vi "Van Der Pauw Test.vi"(8 "error in (no error)":errorcluster) -> (0 "error out":errorcluster)   [LabVIEW 2016, in "Hall Effect Library.lvlib"]
doc: "This VI executes the Van Der Pauw Resisitivty Test and returns the voltage measurements V1-V8 taken during the test."
uses:
  Hall Effect Library.lvlib
  Controls/Measurement.ctl
  Public/Controls/Data Items.ctl
  Public/Controls/Tests.ctl
  Global Variables/Test Settings.vi
  Global Variables/Instrument Locations.vi
  Global Variables/Hall Effect Data.vi
panel:
  out "Soak Until":timestamp
  out "Measurement":T1
  out "Test Step":T2(ring)
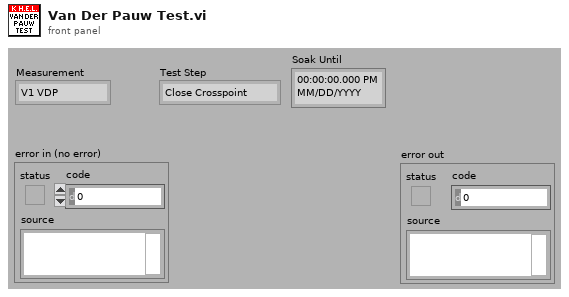
[diagram p1: front panel]
types:
  T1 = typedef "Hall Effect Library.lvlib/Measurement.ctl" = enum16{"V1 VDP", "V2 VDP", "V3 VDP", "V4 VDP", "V5 VDP", "V6 VDP", "V7 VDP", "V8 VDP", "V1 HE", "V2 HE", "V3 HE", "V4 HE", "V5 HE", "V6 HE", "V7 HE", "V8 HE", "V1 Res Bar", "V1 Hall Bar", "V1 Res 6-Cot", "V2 Res 6-Cot", "V3 Res 6-Cot", "V4 Res 6-Cot", "V1 Hall 6-Cot", "V2 Hall 6-Cot", "V3 Hall 6-Cot", "V4 Hall 6-Cot", "V5 Hall 6-Cot", "V6 Hall 6-Cot", "V7 Hall 6-Cot", "V8 Hall 6-Cot", "V1 Res 8-Cot", "V2 Res 8-Cot", "V3 Res 8-Cot", "V4 Res 8-Cot", "V1 Hall 8-Cot", "V2 Hall 8-Cot", "V3 Hall 8-Cot", "V4 Hall 8-Cot"}
  T2 = enum16{"Close Crosspoint", "Soak 1", "Zero Ammeter", "Zero Voltmeter", "I-SRC On", "Init Ammeter", "Soak 2", "Measure I", "Measure V", "I-SRC Off", "Open Crosspoint", "Done"}
  T3 = cluster{"fA":dbl, "fB":dbl, "QA":dbl, "QB":dbl, "pAvg":dbl, "pA":dbl, "pB":dbl}
  T4 = typedef "Hall Effect Library.lvlib/Resisitivity.ctl" = enum16{"Low", "High"}
  T5 = typedef "Hall Effect Library.lvlib/Tests.ctl" = enum16{"Van Der Pauw", "Hall Effect", "Bar Sample Resistivity", "Bar Sample Hall ", "6-Contact Sample Resistivity", "6-Contact Sample Hall", "8-Contact Sample Resistivity", "8-Contact Sample Hall", ""}
  T6 = typedef "Hall Effect Library.lvlib/Data Items.ctl" = enum16{"V1 Van Der Pauw", "V2 Van Der Pauw", "V3 Van Der Pauw", "V4 Van Der Pauw", "V5 Van Der Pauw", "V6 Van Der Pauw", "V7 Van Der Pauw", "V8 Van Der Pauw", "V1 Hall Effect", "V2 Hall Effect", "V3 Hall Effect", "V4 Hall Effect", "V5 Hall Effect", "V6  Hall Effect", "V7 Hall Effect", "V8 Hall Effect", "V1 Res Bar", "V1 Hall Bar", "V1 Res 6-Cot", "V2 Res 6-Cot", "V3 Res 6-Cot", "V4 Res 6-Cot", "V1 Hall 6-Cot", "V2 Hall 6-Cot", "V3 Hall 6-Cot", "V4 Hall 6-Cot", "V5 Hall 6-Cot", "V6 Hall 6-Cot", "V7 Hall 6-Cot", "V8 Hall 6-Cot", "V1 Res 8-Cot", "V2 Res 8-Cot", "V3 Res 8-Cot", "V4 Res 8-Cot", "V1 Hall 8-Cot", "V2 Hall 8-Cot", "V3 Hall 8-Cot", "V4 Hall 8-Cot", "Van Der Pauw Results", "Hall Effect Results", "Bar Sample Resistivity Results", "Bar Sample Hall Results", "6-Contact Resistivity Results", "6-Contact Hall Results", "8-Contact Resistivity Results", "8-Contact Hall Results"}
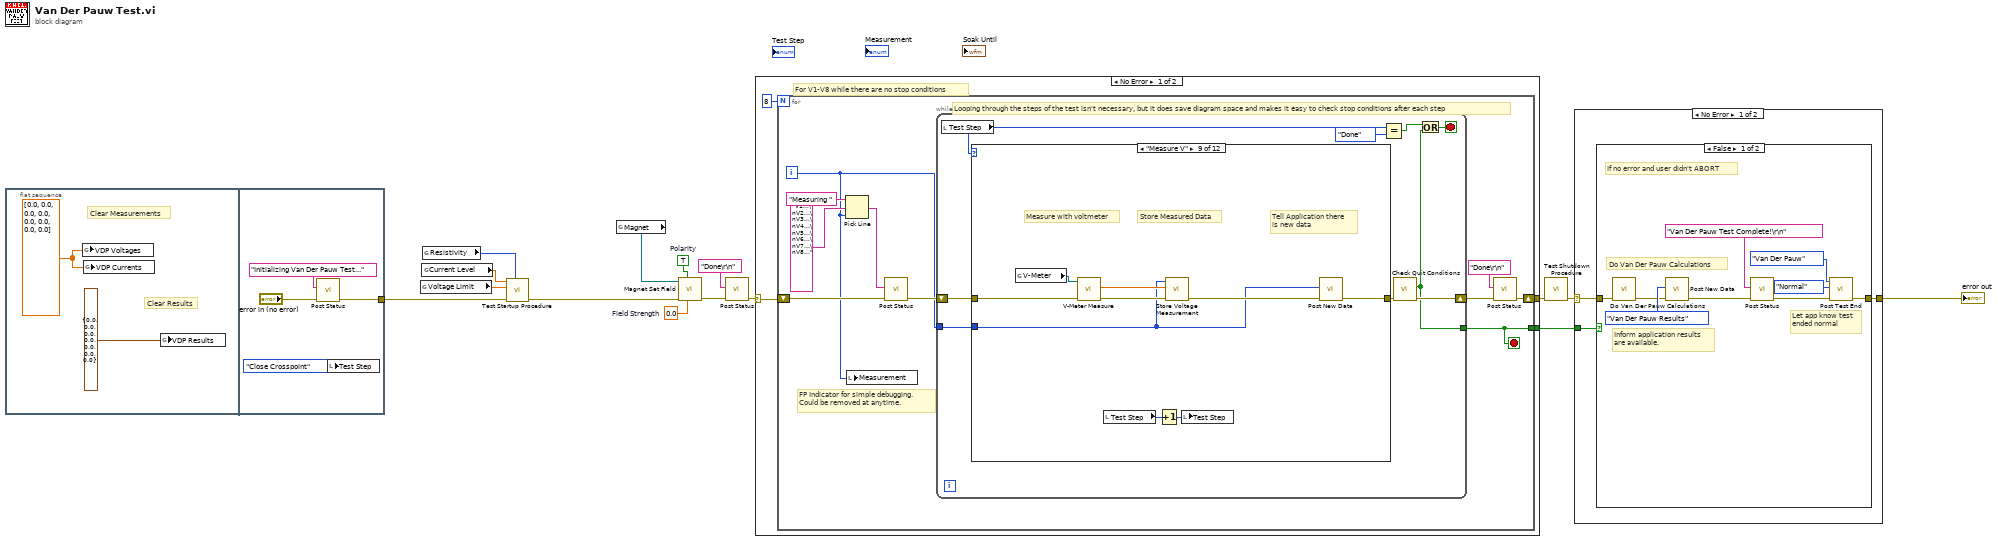
[diagram p0: block diagram]
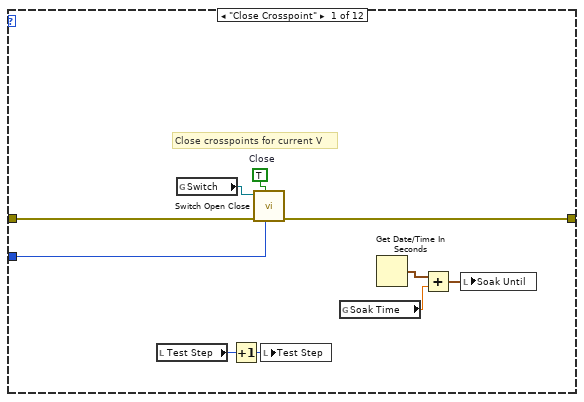
[diagram p2: hidden frame]
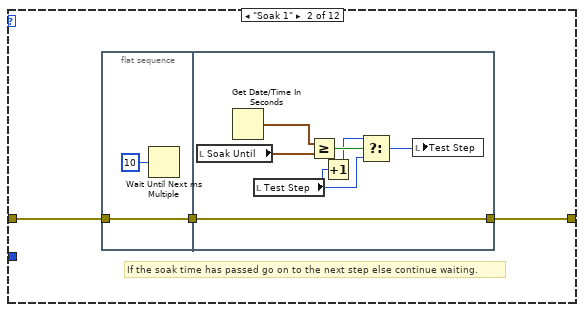
[diagram p3: hidden frame]
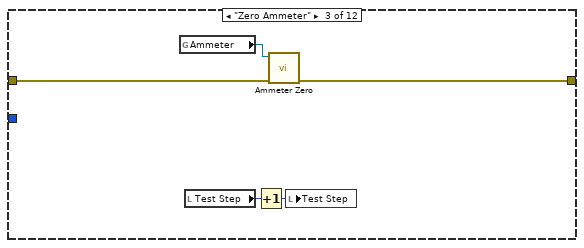
[diagram p4: hidden frame]
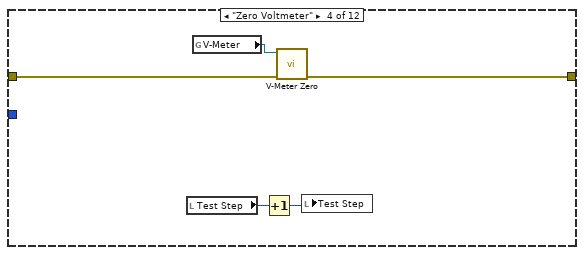
[diagram p5: hidden frame]
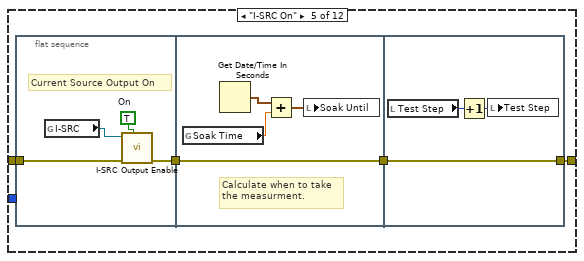
[diagram p6: hidden frame]
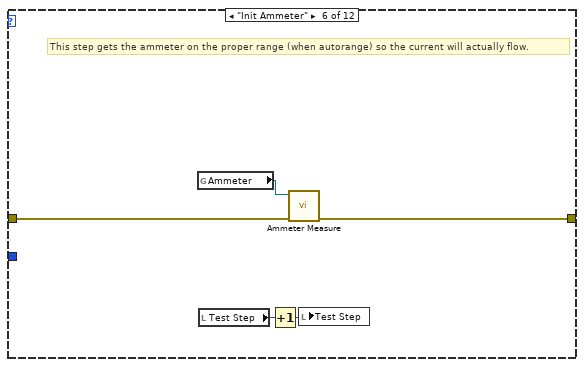
[diagram p7: hidden frame]
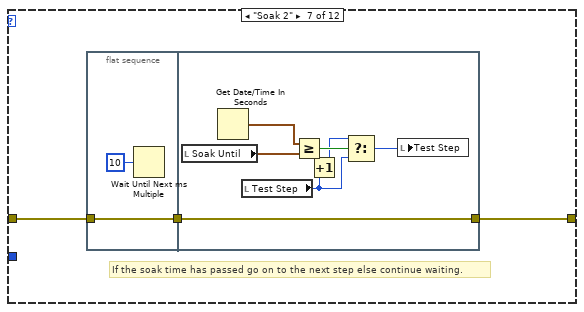
[diagram p8: hidden frame]
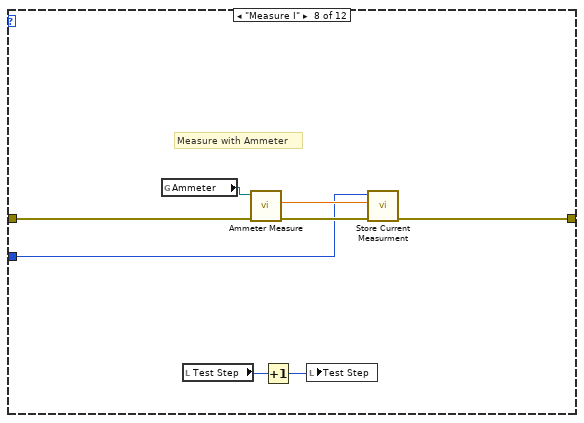
[diagram p9: hidden frame]
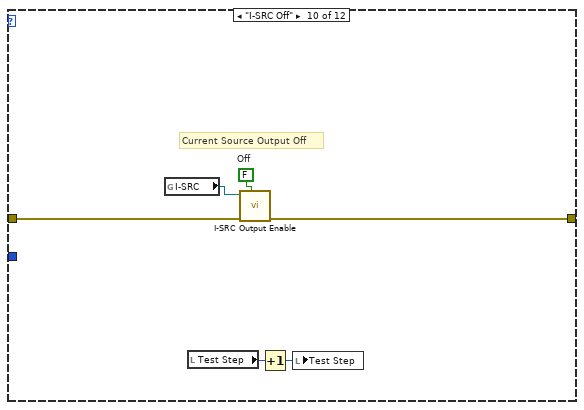
[diagram p10: hidden frame]
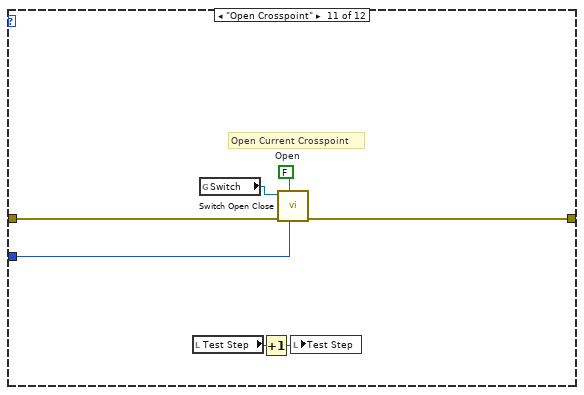
[diagram p11: hidden frame]
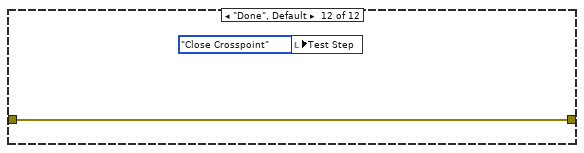
[diagram p12: hidden frame]
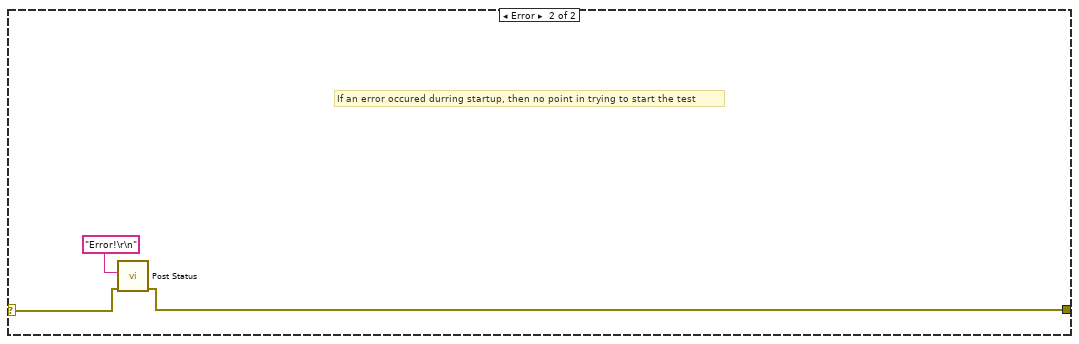
[diagram p13: hidden frame]
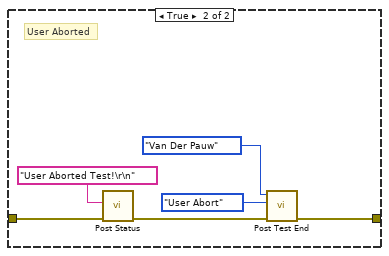
[diagram p14: hidden frame]
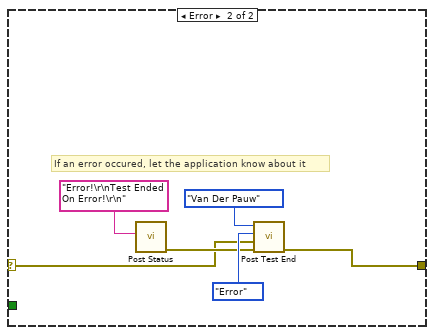
[diagram p15: hidden frame]
diagram:
  w5 = TRUE  # Polarity
  w6 = 0.0  # Field Strength
  n1 = flat-sequence {
    tunnel: [w18] -> w8
    frame #0 {
      w17 = dbl[] [0.0, 0.0, 0.0, 0.0, 0.0, 0.0, 0.0, 0.0] ("Van Der Pauw Voltages")
      # "Clear Results"
      # "Clear Measurements"
      n2 = global write "Hall Effect Data.vi" "VDP Voltages"(w17) -> ()
      n3 = global write "Hall Effect Data.vi" "VDP Currents"(w17) -> ()
      n4 = global write "Hall Effect Data.vi" "VDP Results"(T3 {"fA"=0.0, "fB"=0.0, "QA"=0.0, "QB"=0.0, "pAvg"=0.0, "pA"=0.0, "pB"=0.0} ("Van Der Pauw Results")) -> ()
    }
    frame #1 {
      n5 = call "Post Status.vi"("error in (no error)"="error in (no error)", "Status Message"="Initializing Van Der Pauw Test...") -> ("error out"=w18:errorcluster)  [unwired: 9 out]
      n6 = local write "Test Step"(T2."Close Crosspoint" ("Test Step")) -> ()
    }
  }
  n7 = global read "Test Settings.vi" "Voltage Limit"() -> (w9:dbl)
  n8 = global read "Test Settings.vi" "Current Level"() -> (w10:dbl)
  n9 = global read "Test Settings.vi" "Resistivity"() -> (w11:T4)
  n10 = call "Test Startup Procedure.vi"("Resistivity"=w11, "error in (no error)"=w8, "Voltage Limit"=w9, "Current Level"=w10) -> ("error out"=w2:errorcluster)  [unwired: 7 out]
  n11 = global read "Instrument Locations.vi" "Magnet"() -> (w4:refnum<visa-resource-name>)
  n12 = call "Magnet Set Field.vi"("Field Strength"=w6, "Polarity"=w5, "error in (no error)"=w2, "VISA resource name in"=w4) -> ("error out"=w3:errorcluster)  [unwired: 7 out]
  n13 = call "Post Status.vi"("error in (no error)"=w3, "Status Message"="Done\r\n") -> ("error out"=w1:errorcluster)  [unwired: 9 out]
  n14 = case shown="No Error" w1 {
    selector: w1 -> [w22 w141]
    tunnel: [w25 w142] -> w12
    tunnel: [w24 _] -> w13
    frame No Error {
      # "For V1-V8 while there are no stop conditions"
      n15 = for {
        N: 8 -> [_]
        shift-right: [w28] -> w25
        shift-left: w22 -> [w31]
        tunnel: [w26] -> w24
        i -> [w27]
        stop <- w26 stop-if-true
        # "FP Indicator for simple debugging.\nCould be removed at anytime."
        # "Looping through the steps of the test isn't necessary, but it does save diagram space and makes it easy to check stop conditions after each step"
        n16 = Pick Line(string ("")="Measuring ", multi-line string="V1...\nV2...\nV3...\nV4...\nV5...\nV6...\nV7...\nV8...", line index=w27) -> (output string=w33:string)
        n17 = local write "Measurement"(w27) -> ()
        n18 = call "Post Status.vi"("error in (no error)"=w31, "Status Message"=w33) -> ("error out"=w32:errorcluster)  [unwired: 9 out]
        n19 = while {
          shift-right: [w42] -> w29
          shift-left: w32 -> [w44]
          tunnel: w27 -> [w43]
          tunnel: [w38] -> w26
          stop <- w41 stop-if-true
          n20 = local read "Test Step"() -> (w39:T2)
          n21 = case shown="\"Measure V\"" w39 {
            tunnel: [w52 w55 w69 w74 w79 w95 w98 w113 w120 w128 w136 w140] -> w37
            tunnel: w44 -> [w51 w56 w70 w75 w80 w96 w99 w115 w124 w129 w135 w140]
            tunnel: w43 -> [w50 _ _ _ _ _ _ w111 w119 _ w134 _]
            frame "Close Crosspoint" {
              w53 = TRUE  # Close
              # "Close crosspoints for current V"
              n22 = local read "Test Step"() -> (w46:T2)
              n23 = global read "Instrument Locations.vi" "Switch"() -> (w54:refnum<visa-resource-name>)
              n24 = Increment(x=w46) -> (x+1=w45:T2)
              n25 = call "Switch Open Close.vi"("Measurement"=w50, "Open/Close (F: Open)"=w53, "error in (no error)"=w51, "VISA resource name in"=w54) -> ("error out"=w52:errorcluster)  [unwired: 7 out]
              n26 = local write "Test Step"(w45) -> ()
              n27 = global read "Test Settings.vi" "Soak Time"() -> (w48:dbl)
              n28 = Get Date/Time In Seconds() -> (seconds since 1Jan1904=w47:timestamp)
              n29 = Add(x=w47, y=w48) -> (x+y=w49:timestamp)
              n30 = local write "Soak Until"(w49) -> ()
            }
            frame "Soak 1" {
              # "If the soak time has passed go on to the next step else continue waiting."
              n31 = flat-sequence {
                tunnel: w56 -> [w58]
                tunnel: [w58] -> w57
                tunnel: [w62] -> w55
                tunnel: w57 -> [w62]
                frame #0 {
                  n32 = Wait Until Next ms Multiple(millisecond multiple=u32 10) -> ()  [unwired: 1 out]
                }
                frame #1 {
                  n33 = local read "Soak Until"() -> (w65:timestamp)
                  n34 = Get Date/Time In Seconds() -> (seconds since 1Jan1904=w66:timestamp)
                  n35 = local read "Test Step"() -> (w61:T2)
                  n36 = Greater Or Equal?(x=w66, y=w65) -> (x >= y?=w64:bool)
                  n37 = Increment(x=w61) -> (x+1=w60:T2)
                  n38 = Select(t=w60, s=w64, f=w61) -> (s? t:f=w63:T2)
                  n39 = local write "Test Step"(w63) -> ()
                }
              }
            }
            frame "Zero Ammeter" {
              n40 = global read "Instrument Locations.vi" "Ammeter"() -> (w71:refnum<visa-resource-name>)
              n41 = local read "Test Step"() -> (w68:T2)
              n42 = Increment(x=w68) -> (x+1=w67:T2)
              n43 = call "Ammeter Zero.vi"("error in (no error)"=w70, "VISA resource name in"=w71) -> ("error out"=w69:errorcluster)  [unwired: 9 out]
              n44 = local write "Test Step"(w67) -> ()
            }
            frame "Zero Voltmeter" {
              n45 = local read "Test Step"() -> (w72:T2)
              n46 = global read "Instrument Locations.vi" "V-Meter"() -> (w76:refnum<visa-resource-name>)
              n47 = Increment(x=w72) -> (x+1=w73:T2)
              n48 = call "V-Meter Zero.vi"("error in (no error)"=w75, "VISA resource name in"=w76) -> ("error out"=w74:errorcluster)  [unwired: 9 out]
              n49 = local write "Test Step"(w73) -> ()
            }
            frame "I-SRC On" {
              n50 = flat-sequence {
                tunnel: w80 -> [w82]
                tunnel: [w81] -> w78
                tunnel: w78 -> [w88]
                tunnel: [w88] -> w77
                tunnel: [w91] -> w79
                tunnel: w77 -> [w91]
                frame #0 {
                  w83 = TRUE  # On
                  # "Current Source Output On"
                  n51 = global read "Instrument Locations.vi" "I-SRC"() -> (w84:refnum<visa-resource-name>)
                  n52 = call "I-SRC Output Enable.vi"("Output (Off)"=w83, "error in (no error)"=w82, "VISA resource name in"=w84) -> ("error out"=w81:errorcluster)  [unwired: 8 out]
                }
                frame #1 {
                  # "Calculate when to take\nthe measurment."
                  n53 = global read "Test Settings.vi" "Soak Time"() -> (w86:dbl)
                  n54 = Get Date/Time In Seconds() -> (seconds since 1Jan1904=w85:timestamp)
                  n55 = Add(x=w85, y=w86) -> (x+y=w87:timestamp)
                  n56 = local write "Soak Until"(w87) -> ()
                }
                frame #2 {
                  n57 = local read "Test Step"() -> (w90:T2)
                  n58 = Increment(x=w90) -> (x+1=w89:T2)
                  n59 = local write "Test Step"(w89) -> ()
                }
              }
            }
            frame "Init Ammeter" {
              # "This step gets the ammeter on the proper range (when autorange) so the current will actually flow."
              n60 = global read "Instrument Locations.vi" "Ammeter"() -> (w94:refnum<visa-resource-name>)
              n61 = local read "Test Step"() -> (w93:T2)
              n62 = Increment(x=w93) -> (x+1=w92:T2)
              n63 = call "Ammeter Measure.vi"("error in (no error)"=w96, "VISA resource name in"=w94) -> ("error out"=w95:errorcluster)  [unwired: 9 out]
              n64 = local write "Test Step"(w92) -> ()
            }
            frame "Soak 2" {
              # "If the soak time has passed go on to the next step else continue waiting."
              n65 = flat-sequence {
                tunnel: w99 -> [w100]
                tunnel: [w100] -> w97
                tunnel: [w104] -> w98
                tunnel: w97 -> [w104]
                frame #0 {
                  n66 = Wait Until Next ms Multiple(millisecond multiple=u32 10) -> ()  [unwired: 1 out]
                }
                frame #1 {
                  n67 = local read "Soak Until"() -> (w107:timestamp)
                  n68 = Get Date/Time In Seconds() -> (seconds since 1Jan1904=w108:timestamp)
                  n69 = local read "Test Step"() -> (w102:T2)
                  n70 = Greater Or Equal?(x=w108, y=w107) -> (x >= y?=w106:bool)
                  n71 = Increment(x=w102) -> (x+1=w103:T2)
                  n72 = Select(t=w103, s=w106, f=w102) -> (s? t:f=w105:T2)
                  n73 = local write "Test Step"(w105) -> ()
                }
              }
            }
            frame "Measure I" {
              # "Measure with Ammeter"
              n74 = global read "Instrument Locations.vi" "Ammeter"() -> (w116:refnum<visa-resource-name>)
              n75 = local read "Test Step"() -> (w110:T2)
              n76 = call "Ammeter Measure.vi"("error in (no error)"=w115, "VISA resource name in"=w116) -> ("error out"=w114:errorcluster, "Measurement"=w112:dbl)  [unwired: 8 out]
              n77 = Increment(x=w110) -> (x+1=w109:T2)
              n78 = local write "Test Step"(w109) -> ()
              n79 = call "Store Current Measurment.vi"("error in"=w114, "Value"=w112, "Measurement"=w111) -> ("error out"=w113:errorcluster)  [unwired: 8 out]
            }
            frame "Measure V" {
              # "Tell Application there\nis new data"
              # "Store Measured Data"
              # "Measure with voltmeter"
              n80 = global read "Instrument Locations.vi" "V-Meter"() -> (w125:refnum<visa-resource-name>)
              n81 = call "V-Meter Measure.vi"("error in (no error)"=w124, "VISA resource name in"=w125) -> ("error out"=w123:errorcluster, "Measurement"=w122:dbl)  [unwired: 1 in, 7 out]
              n82 = local read "Test Step"() -> (w118:T2)
              n83 = Increment(x=w118) -> (x+1=w117:T2)
              n84 = call "Store Voltage Measurement.vi"("error in"=w123, "Value"=w122, "Measurement"=w119) -> ("error out"=w121:errorcluster)  [unwired: 8 out]
              n85 = local write "Test Step"(w117) -> ()
              n86 = call "Post New Data.vi"("error in (no error)"=w121, "Data Item"=w119) -> ("error out"=w120:errorcluster)  [unwired: 9 out]
            }
            frame "I-SRC Off" {
              w130 = FALSE  # Off
              # "Current Source Output Off"
              n87 = global read "Instrument Locations.vi" "I-SRC"() -> (w131:refnum<visa-resource-name>)
              n88 = local read "Test Step"() -> (w127:T2)
              n89 = call "I-SRC Output Enable.vi"("Output (Off)"=w130, "error in (no error)"=w129, "VISA resource name in"=w131) -> ("error out"=w128:errorcluster)  [unwired: 8 out]
              n90 = Increment(x=w127) -> (x+1=w126:T2)
              n91 = local write "Test Step"(w126) -> ()
            }
            frame "Open Crosspoint" {
              w137 = FALSE  # Open
              # "Open Current Crosspoint"
              n92 = local read "Test Step"() -> (w132:T2)
              n93 = global read "Instrument Locations.vi" "Switch"() -> (w138:refnum<visa-resource-name>)
              n94 = Increment(x=w132) -> (x+1=w133:T2)
              n95 = call "Switch Open Close.vi"("Measurement"=w134, "Open/Close (F: Open)"=w137, "error in (no error)"=w135, "VISA resource name in"=w138) -> ("error out"=w136:errorcluster)  [unwired: 7 out]
              n96 = local write "Test Step"(w133) -> ()
            }
            frame "Done", Default {
              n97 = local write "Test Step"(T2."Close Crosspoint" ("Test Step")) -> ()
            }
          }
          n98 = Equal?(x=w39, y=T2."Done") -> (x = y?=w40:bool)
          n99 = call "Check Quit Conditions.vi"("error in (no error)"=w37) -> ("error out"=w42:errorcluster, "Quit?"=w38:bool)  [unwired: 9 out]
          n100 = Or(x=w40, y=w38) -> (x .or. y?=w41:bool)
        }
        n101 = call "Post Status.vi"("error in (no error)"=w29, "Status Message"="Done\r\n") -> ("error out"=w28:errorcluster)  [unwired: 9 out]
      }
    }
    frame Error {
      # "If an error occured durring startup, then no point in trying to start the test"
      n102 = call "Post Status.vi"("error in (no error)"=w141, "Status Message"="Error!\r\n") -> ("error out"=w142:errorcluster)  [unwired: 9 out]
    }
  }
  n103 = call "Test Shutdown Procedure.vi"("error in (no error)"=w12) -> ("error out"=w14:errorcluster)  [unwired: 10 out]
  n104 = case shown="No Error" w14 {
    selector: w14 -> [w145 w163]
    tunnel: w13 -> [w146 _]
    tunnel: [w144 w165] -> w15
    frame No Error {
      n105 = case shown="False" w146 {
        tunnel: w145 -> [w154 w160]
        tunnel: [w149 w157] -> w144
        frame False {
          # "Let app know test\nended normal"
          # "Inform application results\nare available."
          # "Do Van Der Pauw Calculations"
          # "If no error and user didn't ABORT"
          n106 = call "Do Van Der Pauw Calculations.vi"("error in (no error)"=w154) -> ("error out"=w153:errorcluster)  [unwired: 10 out]
          n107 = call "Post New Data.vi"("error in (no error)"=w153, "Data Item"=Data_Items."Van Der Pauw Results") -> ("error out"=w151:errorcluster)  [unwired: 9 out]
          n108 = call "Post Status.vi"("error in (no error)"=w151, "Status Message"="Van Der Pauw Test Complete!\r\n") -> ("error out"=w148:errorcluster)  [unwired: 9 out]
          n109 = call "Post Test End.vi"("error in (no error)"=w148, "Test End"=enum16{"Normal", "User Abort", "Error"}."Normal", "Test"=Tests."Van Der Pauw") -> ("error out"=w149:errorcluster)  [unwired: 1 in, 7 out]
        }
        frame True {
          # "User Aborted"
          n110 = call "Post Status.vi"("error in (no error)"=w160, "Status Message"="User Aborted Test!\r\n") -> ("error out"=w159:errorcluster)  [unwired: 9 out]
          n111 = call "Post Test End.vi"("error in (no error)"=w159, "Test End"=enum16{"Normal", "User Abort", "Error"}."User Abort", "Test"=Tests."Van Der Pauw") -> ("error out"=w157:errorcluster)  [unwired: 1 in, 7 out]
        }
      }
    }
    frame Error {
      # "If an error occured, let the application know about it"
      n112 = call "Post Status.vi"("Status Message"="Error!\r\nTest Ended On Error!\r\n") -> ("error out"=w164:errorcluster)  [unwired: 1 in, 9 out]
      n113 = call "Post Test End.vi"("error in (no error)"=w164, "Test End Error (no error)"=w163, "Test End"=enum16{"Normal", "User Abort", "Error"}."Error", "Test"=Tests."Van Der Pauw") -> ("error out"=w165:errorcluster)  [unwired: 7 out]
    }
  }
  "error out" <- w15
